vi "TemperatureReadout.vi"(0 "Handle In":i32, 1 "TC1 +Channel":u16, 2 "TC1 -Channel":u16, 3 "TC2 +Channel":u16, 4 "TC2 -Channel":u16, 5 "error in":errorcluster, 6 "TC1 Type":u16(ring) items=["B", "E", "J", "K", "N", "R", "S", "T"], 7 "TC2 Type":u16(ring) items=["B", "E", "J", "K", "N", "R", "S", "T"]) -> (8 "TC1 Raw Readings":dbl format="%.6f", 9 "TC2 Raw Readings":dbl format="%.6f", 10 "TC1 Temperature (Deg F)":dbl format="%.2f", 11 "TC2 Temperature (Deg F)":dbl format="%.2f", 12 "TC1 Temperature (Deg C)":dbl format="%.2f", 13 "TC2 Temperature (Deg C)":dbl format="%.2f", 15 "TC1 Temperature (Kelvin)":dbl format="%.2f", 18 "TC2 Temperature (Kelvin)":dbl format="%.2f", 19 "error out":errorcluster[](array[cluster]))   [LabVIEW 2021]
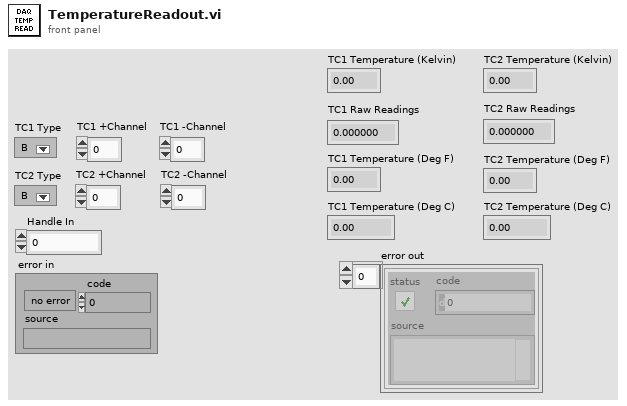
[diagram p1: front panel]
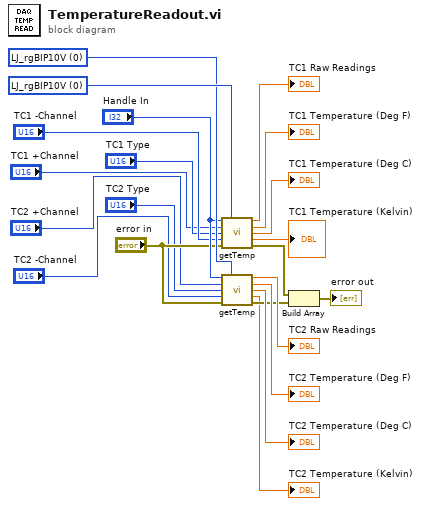
[diagram p0: block diagram]
diagram:
  w20 = u16 0 items=["LJ_rgBIP10V", "LJ_rgBIP1V", "LJ_rgBIPP1V", "LJ_rgBIPP01V"] ("AIN Range")
  w21 = u16 0 items=["LJ_rgBIP10V", "LJ_rgBIP1V", "LJ_rgBIPP1V", "LJ_rgBIPP01V"] ("AIN Range")
  n1 = call "getTemp.vi"("Handle In"="Handle In", "AIN Range"=w21, "+Channel"="TC1 +Channel", "Thermocouple Type"="TC1 Type", "-Channel"="TC1 -Channel", "error in"="error in") -> ("Raw Readings"=→"TC1 Raw Readings":dbl, "Temperature (Deg F)"=→"TC1 Temperature (Deg F)":dbl, "Temperature (Deg C)"=→"TC1 Temperature (Deg C)":dbl, "Temperature (Kelvin)"=→"TC1 Temperature (Kelvin)":dbl, "error out"=w10:errorcluster)  [unwired: 4 in, 1 out]
  n2 = call "getTemp.vi"("Handle In"="Handle In", "AIN Range"=w20, "+Channel"="TC2 +Channel", "Thermocouple Type"="TC2 Type", "-Channel"="TC2 -Channel", "error in"="error in") -> ("Raw Readings"=→"TC2 Raw Readings":dbl, "Temperature (Deg F)"=→"TC2 Temperature (Deg F)":dbl, "Temperature (Deg C)"=→"TC2 Temperature (Deg C)":dbl, "Temperature (Kelvin)"=→"TC2 Temperature (Kelvin)":dbl, "error out"=w11:errorcluster)  [unwired: 4 in, 1 out]
  n3 = Build Array(w10, w11) -> (→"error out":errorcluster[])
